vi "Empty Sepcific Notifier.vi"(8 "error in (no error)":errorcluster, 10 "ID In":i64[](array[numeric]), 11 "Root Actor in":refnum<class "Root Actor.lvclass">) -> (0 "error out":errorcluster, 3 "Root Actor out":refnum<class "Root Actor.lvclass">)   [LabVIEW 2024, in "Root Actor.lvclass"]
uses:
  Root Actor.lvclass
  Root Actor.lvclass/Root Actor.ctl
  Notifier/Notifier.lvclass
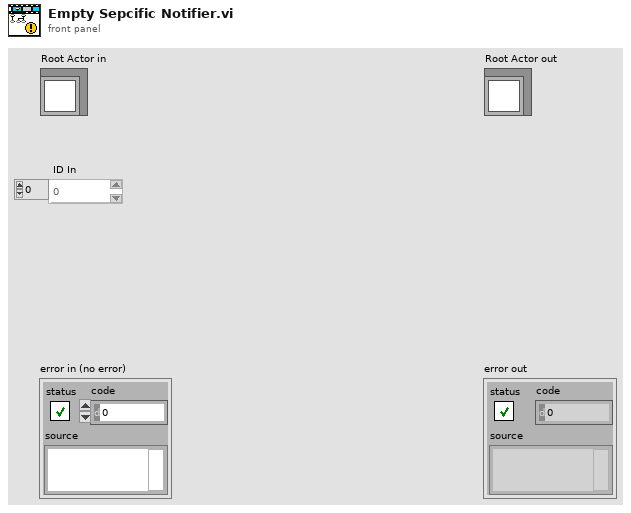
[diagram p1: front panel]
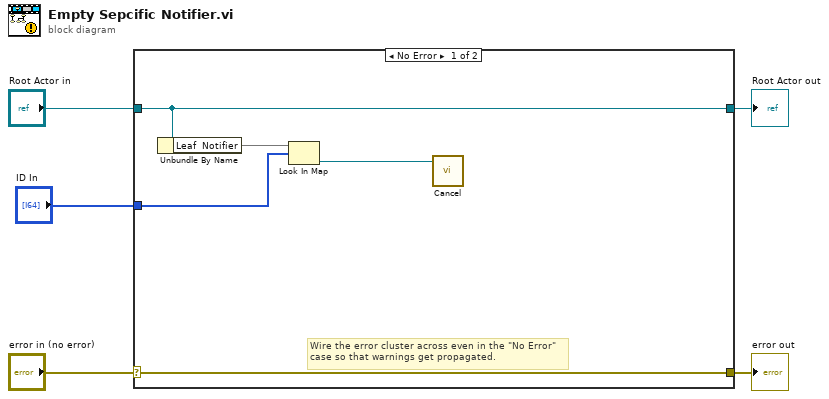
[diagram p0: block diagram]
diagram:
  n1 = case shown="No Error" "error in (no error)" {
    selector: "error in (no error)" -> [w10 w12]
    tunnel: [w10 w12] -> w4
    tunnel: [w9 w11] -> w2
    tunnel: "Root Actor in" -> [w9 w11]
    tunnel: "ID In" -> [w7 _]
    frame No Error {
      # "Wire the error cluster across even in the \"No Error\"\ncase so that warnings get propagated."
      n2 = Unbundle By Name(w9) -> ("Leaf  Notifier"=w8:map{i64[], refnum<class "Notifier.lvclass">})
      n3 = Look In Map(map=w8, key=w7) -> (value=w6:refnum<class "Notifier.lvclass">)  [unwired: 1 in, 1 out]
      n4 = call-dynamic "Cancel.vi"("Notifier in"=w6) -> ()  [unwired: 9 in, 2 out]
    }
    frame Error {
    }
  }
  "error out" <- w4
  "Root Actor out" <- w2
